vi "Cargo Manip Control.vi"   [LabVIEW 2018]
uses:
  SubSystems/Cargo Intake/Cargo Intake Global.vi
  SubSystems/Controllers/Manipulator Controlller/Manipulator Controller Global.vi
  SubSystems/Lift/Lift Global.vi
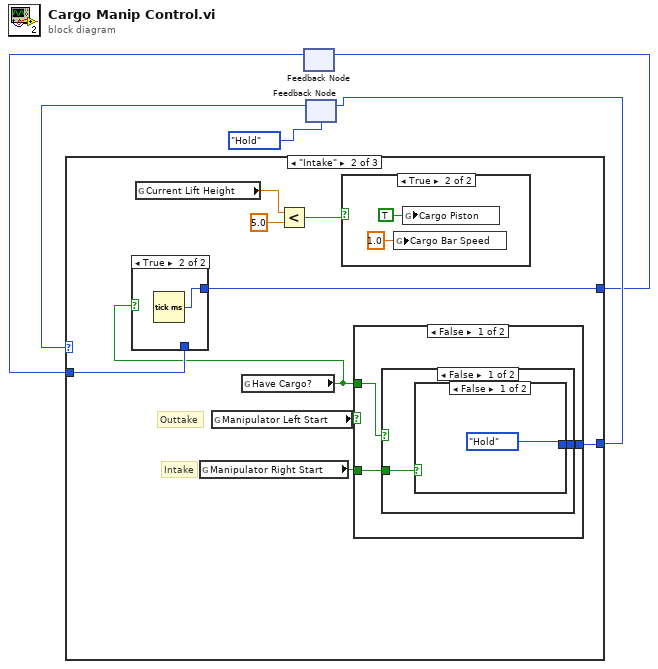
[diagram p0: block diagram]
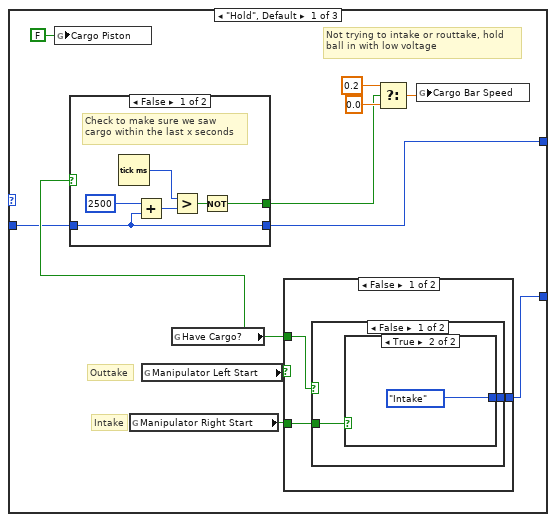
[diagram p2: hidden frame]
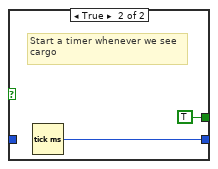
[diagram p3: hidden frame]
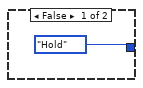
[diagram p4: hidden frame]
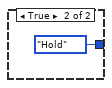
[diagram p5: hidden frame]
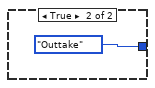
[diagram p6: hidden frame]
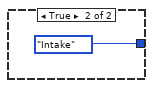
[diagram p9: hidden frame]
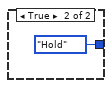
[diagram p10: hidden frame]
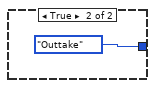
[diagram p11: hidden frame]
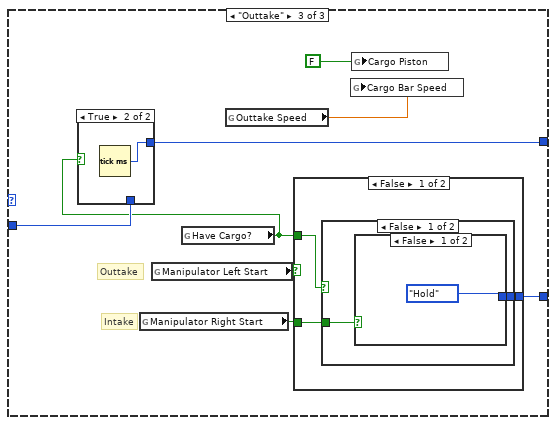
[diagram p12: hidden frame]
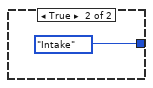
[diagram p14: hidden frame]
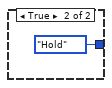
[diagram p15: hidden frame]
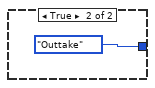
[diagram p16: hidden frame]
diagram:
  n1 = feedback #1() -> (w1:u32)  [unwired: 1 in]
  n2 = feedback #2(enum16{"Going Up", "Outtake", "Intake", "Hold"}."Hold") -> (w4:enum16{"Going Up", "Outtake", "Intake", "Hold"})
  n3 = case shown="\"Intake\"" w4 {
    tunnel: [w14 w40 w61] -> w3
    tunnel: [w9 w38 w59] -> w2
    tunnel: w1 -> [w7 w39 w60]
    frame "Hold", Default {
      # "Outtake"
      # "Intake"
      # "Not trying to intake or routtake, hold\nball in with low voltage"
      n4 = global write "Cargo Intake Global.vi" "Cargo Piston"(FALSE ("Cargo Piston")) -> ()
      n5 = global read "Manipulator Controller Global.vi" "Manipulator Right Start"() -> (w16:bool)
      n6 = global read "Manipulator Controller Global.vi" "Manipulator Left Start"() -> (w15:bool)
      n7 = global read "Cargo Intake Global.vi" "Have Cargo?"() -> (w8:bool)
      n8 = case shown="False" w8 {
        tunnel: [w22 w24] -> w9
        tunnel: w7 -> [w22 _]
        tunnel: [w17 TRUE] -> w6
        frame False {
          # "Check to make sure we saw \ncargo within the last x seconds"
          n9 = Tick Count (ms)() -> (millisecond timer value=w19:u32)
          n10 = Add(x=u32 2500, y=w22) -> (x+y=w20:u32)
          n11 = Greater?(x=w19, y=w20) -> (0:w18:bool)
          n12 = Not(x=w18) -> (.not. x?=w17:bool)
        }
        frame True {
          # "Start a timer whenever we see\ncargo"
          n13 = Tick Count (ms)() -> (millisecond timer value=w24:u32)
        }
      }
      n14 = case shown="False" w15 {
        tunnel: w16 -> [w27 _]
        tunnel: [w26 enum16{"Going Up", "Outtake", "Intake", "Hold"}."Outtake"] -> w14
        tunnel: w8 -> [w25 _]
        frame False {
          n15 = case shown="False" w25 {
            tunnel: w27 -> [w29 _]
            tunnel: [w28 enum16{"Going Up", "Outtake", "Intake", "Hold"}."Hold"] -> w26
            frame False {
              n16 = case shown="True" w29 {
                tunnel: [enum16{"Going Up", "Outtake", "Intake", "Hold"}."Hold" enum16{"Going Up", "Outtake", "Intake", "Hold"}."Intake"] -> w28
                frame False {
                }
                frame True {
                }
              }
            }
            frame True {
            }
          }
        }
        frame True {
        }
      }
      n17 = Select(t=0.2, s=w6, f=0.0) -> (s? t:f=w12:dbl)
      n18 = global write "Cargo Intake Global.vi" "Cargo Bar Speed"(w12) -> ()
    }
    frame "Intake" {
      # "Outtake"
      # "Intake"
      n19 = global read "Lift Global.vi" "Current Lift Height"() -> (w35:dbl)
      n20 = global read "Manipulator Controller Global.vi" "Manipulator Right Start"() -> (w42:bool)
      n21 = global read "Manipulator Controller Global.vi" "Manipulator Left Start"() -> (w41:bool)
      n22 = global read "Cargo Intake Global.vi" "Have Cargo?"() -> (w37:bool)
      n23 = case shown="True" w37 {
        tunnel: w39 -> [w45 _]
        tunnel: [w45 w46] -> w38
        frame False {
        }
        frame True {
          n24 = Tick Count (ms)() -> (millisecond timer value=w46:u32)
        }
      }
      n25 = Less?(x=w35, y=5.0) -> (x < y?=w36:bool)
      n26 = case shown="True" w36 {
        frame False {
        }
        frame True {
          n27 = global write "Cargo Intake Global.vi" "Cargo Bar Speed"(1.0 ("Cargo Bar Speed")) -> ()
          n28 = global write "Cargo Intake Global.vi" "Cargo Piston"(TRUE ("Cargo Piston")) -> ()
        }
      }
      n29 = case shown="False" w41 {
        tunnel: w42 -> [w49 _]
        tunnel: [w48 enum16{"Going Up", "Outtake", "Intake", "Hold"}."Outtake"] -> w40
        tunnel: w37 -> [w47 _]
        frame False {
          n30 = case shown="False" w47 {
            tunnel: w49 -> [w51 _]
            tunnel: [w50 enum16{"Going Up", "Outtake", "Intake", "Hold"}."Hold"] -> w48
            frame False {
              n31 = case shown="False" w51 {
                tunnel: [enum16{"Going Up", "Outtake", "Intake", "Hold"}."Hold" enum16{"Going Up", "Outtake", "Intake", "Hold"}."Intake"] -> w50
                frame False {
                }
                frame True {
                }
              }
            }
            frame True {
            }
          }
        }
        frame True {
        }
      }
    }
    frame "Outtake" {
      # "Outtake"
      # "Intake"
      n32 = global read "Manipulator Controller Global.vi" "Manipulator Right Start"() -> (w63:bool)
      n33 = global read "Manipulator Controller Global.vi" "Manipulator Left Start"() -> (w62:bool)
      n34 = global read "Cargo Intake Global.vi" "Have Cargo?"() -> (w58:bool)
      n35 = case shown="True" w58 {
        tunnel: w60 -> [w64 _]
        tunnel: [w64 w65] -> w59
        frame False {
        }
        frame True {
          n36 = Tick Count (ms)() -> (millisecond timer value=w65:u32)
        }
      }
      n37 = global read "Cargo Intake Global.vi" "Outtake Speed"() -> (w57:dbl)
      n38 = case shown="False" w62 {
        tunnel: w63 -> [w68 _]
        tunnel: [w67 enum16{"Going Up", "Outtake", "Intake", "Hold"}."Outtake"] -> w61
        tunnel: w58 -> [w66 _]
        frame False {
          n39 = case shown="False" w66 {
            tunnel: w68 -> [w70 _]
            tunnel: [w69 enum16{"Going Up", "Outtake", "Intake", "Hold"}."Hold"] -> w67
            frame False {
              n40 = case shown="False" w70 {
                tunnel: [enum16{"Going Up", "Outtake", "Intake", "Hold"}."Hold" enum16{"Going Up", "Outtake", "Intake", "Hold"}."Intake"] -> w69
                frame False {
                }
                frame True {
                }
              }
            }
            frame True {
            }
          }
        }
        frame True {
        }
      }
      n41 = global write "Cargo Intake Global.vi" "Cargo Bar Speed"(w57) -> ()
      n42 = global write "Cargo Intake Global.vi" "Cargo Piston"(FALSE) -> ()
    }
  }
  n43 = feedback-in #1(w2) -> ()
  n44 = feedback-in #2(w3) -> ()
